vi "ThorlabsManager.vi"(3 "error in (no error)":errorcluster caption="错误输入（无错误）", 4 "Input":T3, 5 "ref_in":T1) -> (0 "error out":errorcluster caption="错误输出", 1 "Output":T3, 2 "ref_out":T1)   [LabVIEW 2012]
panel:
  in  "ref_type":T2
  in  "MG17Motor 6":refnum<k7>(container)
  in  "MG17Motor 5":refnum<k7>(container)
  in  "MG17Motor 4":refnum<k7>(container)
  in  "MG17Motor 3":refnum<k7>(container)
  in  "MG17Motor 2":refnum<k7>(container)
  in  "MG17Motor":refnum<k7>(container)
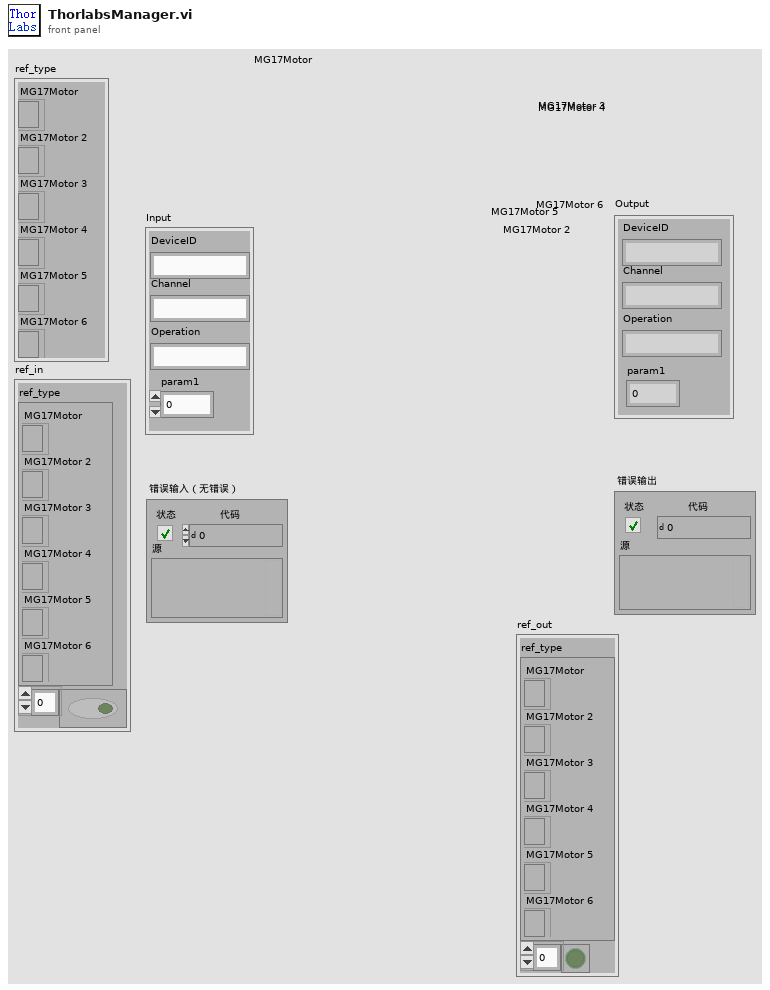
[diagram p1: front panel]
types:
  T1 = cluster{"ref_type":cluster{"MG17Motor":refnum<k7>, "MG17Motor 2":refnum<k7>, "MG17Motor 3":refnum<k7>, "MG17Motor 4":refnum<k7>, "MG17Motor 5":refnum<k7>, "MG17Motor 6":refnum<k7>}, bool[]}
  T2 = cluster{"MG17Motor":refnum<k7>, "MG17Motor 2":refnum<k7>, "MG17Motor 3":refnum<k7>, "MG17Motor 4":refnum<k7>, "MG17Motor 5":refnum<k7>, "MG17Motor 6":refnum<k7>}
  T3 = cluster{"DeviceID":string, "Channel":string, "param1":dbl, "Operation":string}
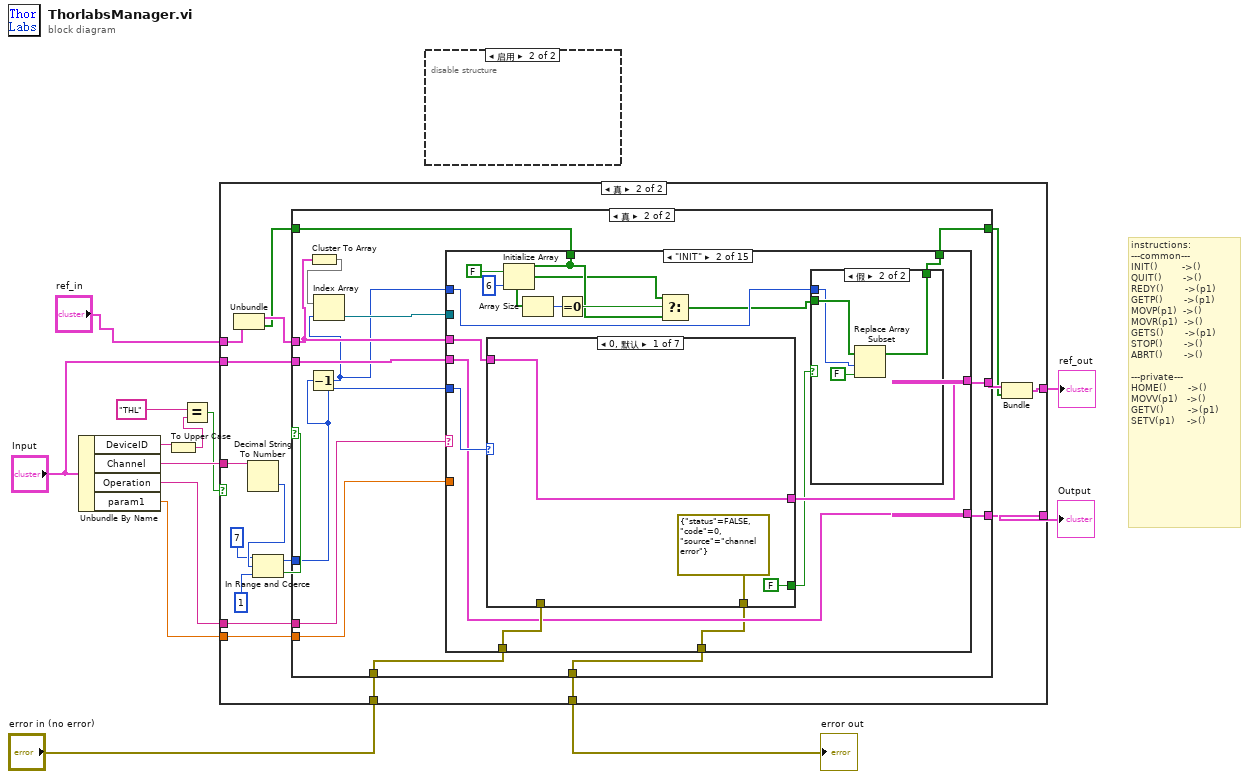
[diagram p0: block diagram]
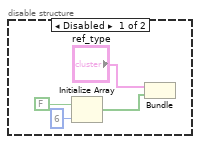
[diagram p2: hidden frame]
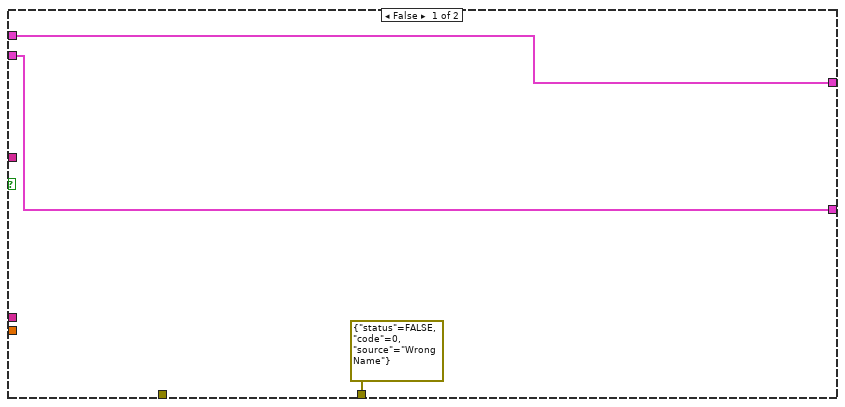
[diagram p3: hidden frame]
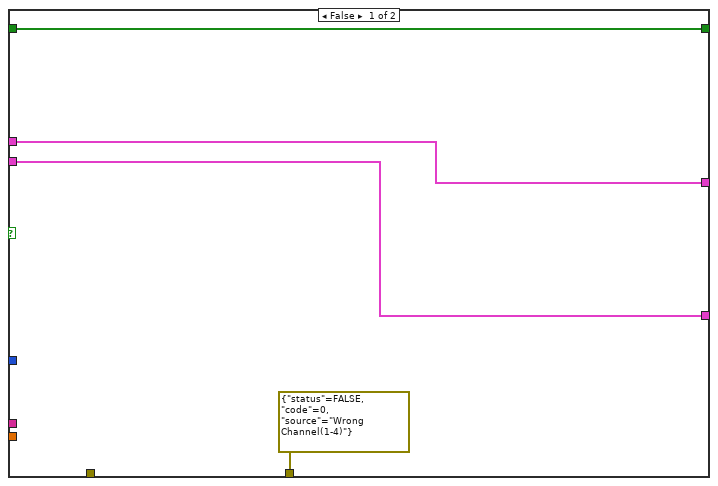
[diagram p4: hidden frame]
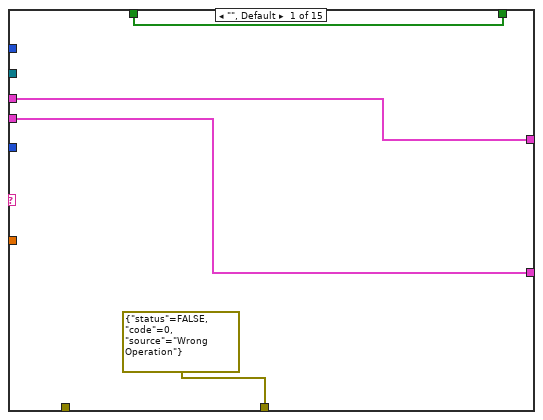
[diagram p5: hidden frame]
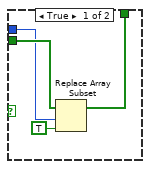
[diagram p6: hidden frame]
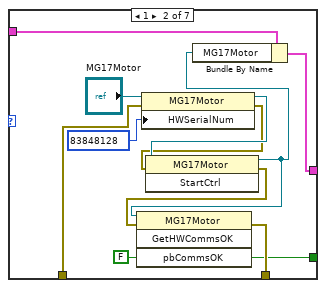
[diagram p7: hidden frame]
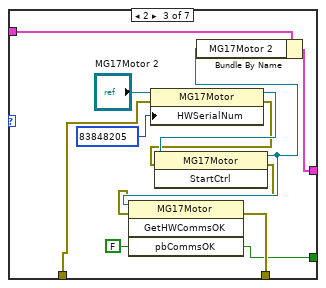
[diagram p8: hidden frame]
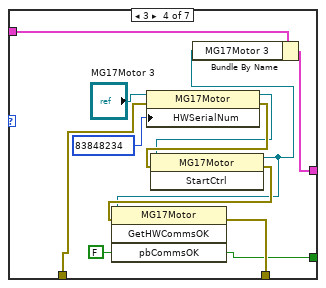
[diagram p9: hidden frame]
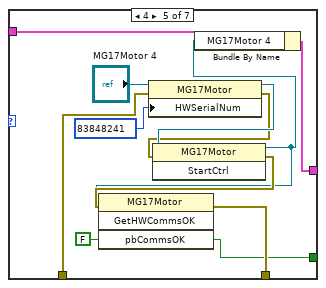
[diagram p10: hidden frame]
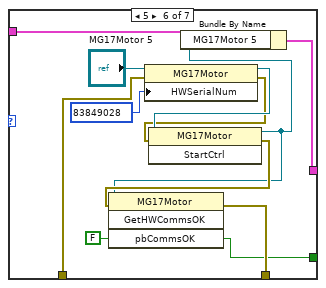
[diagram p11: hidden frame]
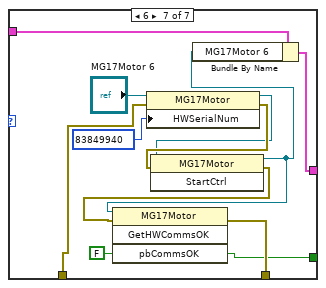
[diagram p12: hidden frame]
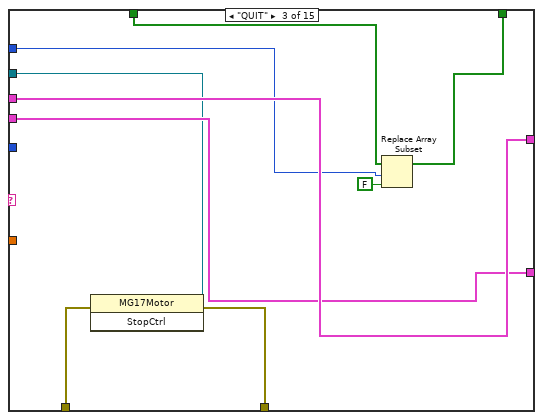
[diagram p13: hidden frame]
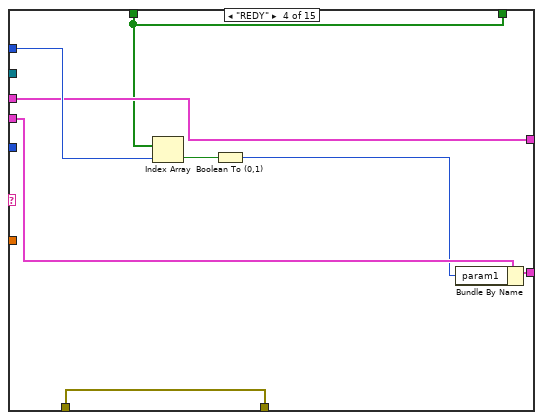
[diagram p14: hidden frame]
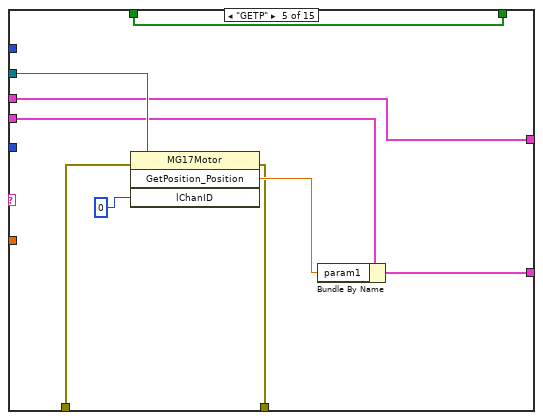
[diagram p15: hidden frame]
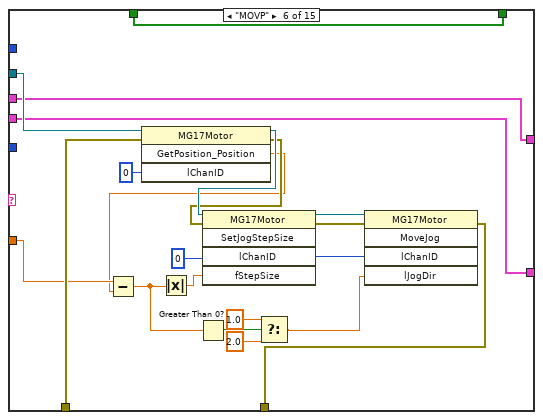
[diagram p16: hidden frame]
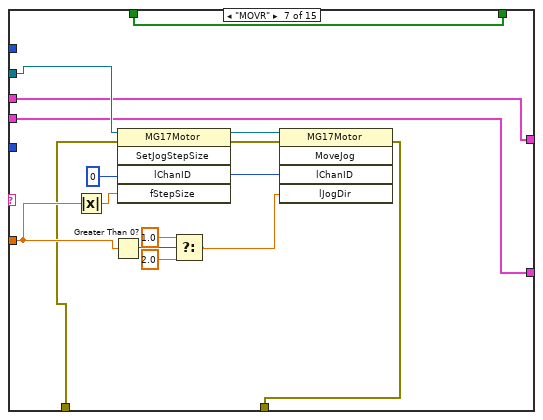
[diagram p17: hidden frame]
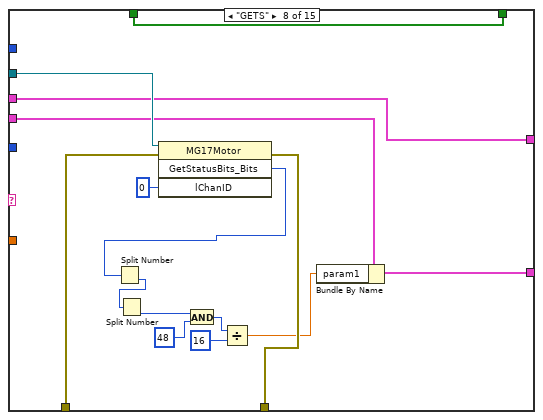
[diagram p18: hidden frame]
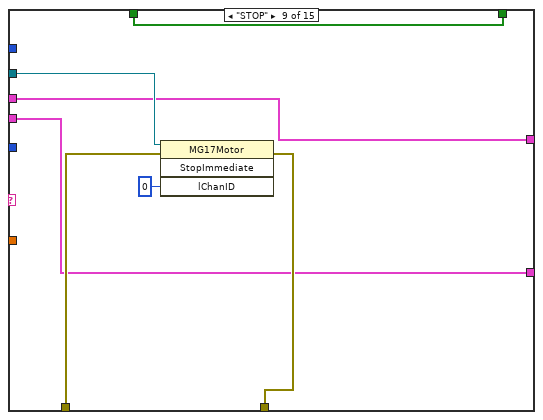
[diagram p19: hidden frame]
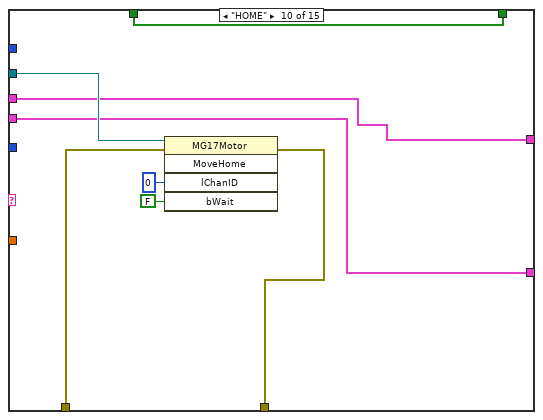
[diagram p20: hidden frame]
diagram:
  # "instructions:\n---common---\nINIT()        ->()\nQUIT()       ->()\nREDY()       ->(p1)\nGETP()       ->(p1)\nMOVP(p1)  ->()\nMOVR(p1)  ->()\nGETS()       ->(p1)\nSTOP()       ->()\nABRT()       ->()\n\n---private---\nHOME()       ->()\nMOVV(p1)   ->()\nGETV()        ->(p1)\nSETV(p1)    ->()"
  n1 = Unbundle By Name("Input") -> ("DeviceID"=w2:string, "Channel"=w12:string, "Operation"=w11:string, "param1"=w10:dbl)
  n2 = To Upper Case(1:w2) -> (0:w1:string)
  n3 = Equal?(x="THL", y=w1) -> (x = y?=w5:bool)
  n4 = case shown="真" w5 {
    tunnel: w12 -> [_ w34]
    tunnel: w11 -> [_ w28]
    tunnel: w10 -> [_ w27]
    tunnel: "error in (no error)" -> [_ w26]
    tunnel: [errorcluster {"status"=FALSE, "code"=0, "source"="Wrong Name"} ("error out") w25] -> w8
    tunnel: [w16 w24] -> w7
    tunnel: "ref_in" -> [w14 w22]
    tunnel: "Input" -> [w16 w23]
    tunnel: [w14 w17] -> w4
    frame False {
    }
    frame True {
      n5 = Unbundle(w22) -> ("ref_type"=w21:T2, w20:bool[])
      n6 = Decimal String To Number(string=w34) -> (number=w33:i32)  [unwired: 2 in, 1 out]
      n7 = In Range and Coerce(upper limit=7 ("上限"), x=w33, lower limit=1 ("下限")) -> (coerced(x)=w29:i32, In Range?=w30:bool)
      n8 = case shown="真" w30 {
        tunnel: w29 -> [_ w42]
        tunnel: w28 -> [_ w52]
        tunnel: w27 -> [_ w51]
        tunnel: w26 -> [_ w50]
        tunnel: [errorcluster {"status"=FALSE, "code"=0, "source"="Wrong Channel(1-4)"} ("error out") w49] -> w25
        tunnel: [w38 w48] -> w24
        tunnel: w21 -> [w36 w45]
        tunnel: w23 -> [w38 w47]
        tunnel: [w36 w46] -> w19
        tunnel: w20 -> [w35 w41]
        tunnel: [w35 w40] -> w18
        frame False {
        }
        frame True {
          n9 = Decrement(x=w42) -> (x-1=w39:i32)
          n10 = Cluster To Array(cluster=w45) -> (array=w44:refnum<k7>[])
          n11 = Index Array(array=w44, index=w39) -> (element=w43:refnum<k7>)
          n12 = case shown="\"INIT\"" w52 {
            tunnel: w42 -> [_ w72 _ _ _ _ _ _ _ _ _ _ _ _ _]
            tunnel: w51 -> [_ _ _ _ _ w189 w213 _ _ _ w253 _ w279 w283 w298]
            tunnel: w50 -> [_ w70 w164 w165 w174 w190 w211 w231 w238 w247 w257 w262 w275 w287 w296]
            tunnel: [errorcluster {"status"=FALSE, "code"=0, "source"="Wrong Operation"} ("error out") w67 w160 w165 w175 w185 w210 w232 w237 w246 w256 w261 w274 w288 w295] -> w49
            tunnel: [w56 w68 w162 w170 w179 w183 w209 w227 w235 w245 w254 w266 w278 w285 w293] -> w48
            tunnel: w45 -> [w54 w71 w163 w167 w177 w184 w208 w228 w236 w244 w255 w263 w277 w286 w294]
            tunnel: w47 -> [w56 w68 w162 w169 w178 w183 w209 w229 w235 w245 w254 w265 w278 w285 w293]
            tunnel: [w54 w69 w163 w167 w177 w184 w208 w228 w236 w244 w255 w263 w277 w286 w294] -> w46
            tunnel: w43 -> [_ _ w161 _ w181 w193 w212 w233 w240 w248 w258 w269 w281 w291 w297]
            tunnel: w41 -> [w53 w62 w158 w166 w173 w182 w207 w219 w234 w242 w260 w267 w276 w284 w292]
            tunnel: [w53 w65 w157 w166 w173 w182 w207 w219 w234 w242 w260 w267 w276 w284 w292] -> w40
            tunnel: w39 -> [_ w66 w159 w172 _ _ _ _ _ _ _ _ _ _ _]
            frame "", Default {
            }
            frame "INIT" {
              n13 = case shown="0, 默认" w72 {
                tunnel: w71 -> [w82 w91 w103 w115 w127 w139 w150]
                tunnel: w70 -> [_ w90 w101 w113 w125 w137 w151]
                tunnel: [errorcluster {"status"=FALSE, "code"=0, "source"="channel error"} ("错误输出") w86 w98 w110 w122 w134 w146] -> w67
                tunnel: [w82 w89 w102 w114 w126 w138 w149] -> w69
                tunnel: [FALSE ("pbCommsOK") w84 w96 w108 w120 w132 w144] -> w57
                frame 0, Default {
                }
                frame 1 {
                  n14 = property class="MG17Motor"(reference="MG17Motor", error in=w90, "HWSerialNum"=83848128) -> (reference out=w94:refnum<k7>, error out=w92:errorcluster)
                  n15 = invoke class="MG17Motor" method="StartCtrl"(reference=w94, error in=w92) -> (reference out=w88:refnum<k7>, error out=w87:errorcluster)  [unwired: 1 in, 1 out]
                  n16 = invoke class="MG17Motor" method="GetHWCommsOK"(reference=w88, error in=w87, "pbCommsOK"=FALSE ("pbStarted")) -> (error out=w86:errorcluster, "pbCommsOK"=w84:bool)  [unwired: 1 in, 2 out]
                  n17 = Bundle By Name(cluster=w91, "MG17Motor"=w88) -> (w89:T2)
                }
                frame 2 {
                  n18 = property class="MG17Motor"(reference="MG17Motor 2", error in=w101, "HWSerialNum"=83848205) -> (reference out=w106:refnum<k7>, error out=w104:errorcluster)
                  n19 = invoke class="MG17Motor" method="StartCtrl"(reference=w106, error in=w104) -> (reference out=w100:refnum<k7>, error out=w99:errorcluster)  [unwired: 1 in, 1 out]
                  n20 = invoke class="MG17Motor" method="GetHWCommsOK"(reference=w100, error in=w99, "pbCommsOK"=FALSE ("pbStarted")) -> (error out=w98:errorcluster, "pbCommsOK"=w96:bool)  [unwired: 1 in, 2 out]
                  n21 = Bundle By Name(cluster=w103, "MG17Motor 2"=w100) -> (w102:T2)
                }
                frame 3 {
                  n22 = property class="MG17Motor"(reference="MG17Motor 3", error in=w113, "HWSerialNum"=83848234) -> (reference out=w117:refnum<k7>, error out=w119:errorcluster)
                  n23 = invoke class="MG17Motor" method="StartCtrl"(reference=w117, error in=w119) -> (reference out=w111:refnum<k7>, error out=w112:errorcluster)  [unwired: 1 in, 1 out]
                  n24 = invoke class="MG17Motor" method="GetHWCommsOK"(reference=w111, error in=w112, "pbCommsOK"=FALSE ("pbStarted")) -> (error out=w110:errorcluster, "pbCommsOK"=w108:bool)  [unwired: 1 in, 2 out]
                  n25 = Bundle By Name(cluster=w115, "MG17Motor 3"=w111) -> (w114:T2)
                }
                frame 4 {
                  n26 = property class="MG17Motor"(reference="MG17Motor 4", error in=w125, "HWSerialNum"=83848241) -> (reference out=w130:refnum<k7>, error out=w128:errorcluster)
                  n27 = invoke class="MG17Motor" method="StartCtrl"(reference=w130, error in=w128) -> (reference out=w123:refnum<k7>, error out=w124:errorcluster)  [unwired: 1 in, 1 out]
                  n28 = invoke class="MG17Motor" method="GetHWCommsOK"(reference=w123, error in=w124, "pbCommsOK"=FALSE ("pbStarted")) -> (error out=w122:errorcluster, "pbCommsOK"=w120:bool)  [unwired: 1 in, 2 out]
                  n29 = Bundle By Name(cluster=w127, "MG17Motor 4"=w123) -> (w126:T2)
                }
                frame 5 {
                  n30 = property class="MG17Motor"(reference="MG17Motor 5", error in=w137, "HWSerialNum"=83849028) -> (reference out=w142:refnum<k7>, error out=w140:errorcluster)
                  n31 = invoke class="MG17Motor" method="StartCtrl"(reference=w142, error in=w140) -> (reference out=w135:refnum<k7>, error out=w136:errorcluster)  [unwired: 1 in, 1 out]
                  n32 = invoke class="MG17Motor" method="GetHWCommsOK"(reference=w135, error in=w136, "pbCommsOK"=FALSE ("pbStarted")) -> (error out=w134:errorcluster, "pbCommsOK"=w132:bool)  [unwired: 1 in, 2 out]
                  n33 = Bundle By Name(cluster=w139, "MG17Motor 5"=w135) -> (w138:T2)
                }
                frame 6 {
                  n34 = property class="MG17Motor"(reference="MG17Motor 6", error in=w151, "HWSerialNum"=83849940) -> (reference out=w153:refnum<k7>, error out=w155:errorcluster)
                  n35 = invoke class="MG17Motor" method="StartCtrl"(reference=w153, error in=w155) -> (reference out=w147:refnum<k7>, error out=w148:errorcluster)  [unwired: 1 in, 1 out]
                  n36 = invoke class="MG17Motor" method="GetHWCommsOK"(reference=w147, error in=w148, "pbCommsOK"=FALSE ("pbStarted")) -> (error out=w146:errorcluster, "pbCommsOK"=w144:bool)  [unwired: 1 in, 2 out]
                  n37 = Bundle By Name(cluster=w150, "MG17Motor 6"=w147) -> (w149:T2)
                }
              }
              n38 = Initialize Array(FALSE, 6 ("维数大小")) -> (w58:bool[])
              n39 = Array Size(array=w62) -> (size(s)=w64:i32)
              n40 = Equal To 0?(x=w64) -> (x = 0?=w63:bool)
              n41 = Select(t=w58, s=w63, f=w62) -> (s? t:f=w61:bool[])
              n42 = case shown="假" w57 {
                tunnel: w61 -> [w76 w79]
                tunnel: w66 -> [w75 w78]
                tunnel: [w73 w77] -> w65
                frame True {
                  n43 = Replace Array Subset(array=w76, new element=TRUE ("新元素/子数组"), index=w75) -> (w73:bool[])
                }
                frame False {
                  n44 = Replace Array Subset(array=w79, new element=FALSE ("新元素/子数组"), index=w78) -> (w77:bool[])
                }
              }
            }
            frame "QUIT" {
              n45 = invoke class="MG17Motor" method="StopCtrl"(reference=w161, error in=w164) -> (error out=w160:errorcluster)  [unwired: 1 in, 2 out]
              n46 = Replace Array Subset(array=w158, new element=FALSE ("新元素/子数组"), index=w159) -> (w157:bool[])
            }
            frame "REDY" {
              n47 = Index Array(array=w166, index=w172) -> (element=w171:bool)
              n48 = Boolean To (0,1)(Boolean=w171) -> (0, 1=w168:i16)
              n49 = Bundle By Name(cluster=w169, "param1"=w168) -> (w170:T3)
            }
            frame "GETP" {
              n50 = invoke class="MG17Motor" method="GetPosition_Position"(reference=w181, error in=w174, "lChanID"=0) -> (error out=w175:errorcluster, "GetPosition_Position"=w176:sgl)  [unwired: 1 in, 2 out]
              n51 = Bundle By Name(cluster=w178, "param1"=w176) -> (w179:T3)
            }
            frame "MOVP" {
              n52 = invoke class="MG17Motor" method="GetPosition_Position"(reference=w193, error in=w190, "lChanID"=0) -> (reference out=w192:refnum<k7>, error out=w191:errorcluster, "GetPosition_Position"=w188:sgl)  [unwired: 1 in, 1 out]
              n53 = Subtract(x=w189, y=w188) -> (x-y=w186:dbl)
              n54 = Absolute Value(x=w186) -> (abs(x)=w195:dbl)
              n55 = Greater Than 0?(x=w186) -> (x > 0?=w199:bool)
              n56 = invoke class="MG17Motor" method="SetJogStepSize"(reference=w192, error in=w191, "lChanID"=0, "fStepSize"=w195) -> (reference out=w198:refnum<k7>, error out=w197:errorcluster, "lChanID"=w196:i32)  [unwired: 1 in, 2 out]
              n57 = Select(t=1.0, s=w199, f=2.0) -> (s? t:f=w200:dbl)
              n58 = invoke class="MG17Motor" method="MoveJog"(reference=w198, error in=w197, "lChanID"=w196, "lJogDir"=w200) -> (error out=w185:errorcluster)  [unwired: 1 in, 4 out]
            }
            frame "MOVR" {
              n59 = Absolute Value(x=w213) -> (abs(x)=w217:dbl)
              n60 = Greater Than 0?(x=w213) -> (x > 0?=w206:bool)
              n61 = invoke class="MG17Motor" method="SetJogStepSize"(reference=w212, error in=w211, "lChanID"=0, "fStepSize"=w217) -> (reference out=w214:refnum<k7>, error out=w215:errorcluster, "lChanID"=w216:i32)  [unwired: 1 in, 2 out]
              n62 = Select(t=1.0, s=w206, f=2.0) -> (s? t:f=w205:dbl)
              n63 = invoke class="MG17Motor" method="MoveJog"(reference=w214, error in=w215, "lChanID"=w216, "lJogDir"=w205) -> (error out=w210:errorcluster)  [unwired: 1 in, 4 out]
            }
            frame "GETS" {
              n64 = invoke class="MG17Motor" method="GetStatusBits_Bits"(reference=w233, error in=w231, "lChanID"=0) -> (error out=w232:errorcluster, "GetStatusBits_Bits"=w226:i32)  [unwired: 1 in, 2 out]
              n65 = Split Number(x=w226) -> (lo(x)=w225:u16)  [unwired: 1 out]
              n66 = Split Number(x=w225) -> (lo(x)=w224:u8)  [unwired: 1 out]
              n67 = And(x=w224, y=u8 48) -> (x .and. y?=w222:u8)
              n68 = Divide(x=w222, y=u8 16) -> (x/y=w220:dbl)
              n69 = Bundle By Name(cluster=w229, "param1"=w220) -> (w227:T3)
            }
            frame "STOP" {
              n70 = invoke class="MG17Motor" method="StopImmediate"(reference=w240, error in=w238, "lChanID"=0) -> (error out=w237:errorcluster)  [unwired: 1 in, 3 out]
            }
            frame "HOME" {
              n71 = invoke class="MG17Motor" method="MoveHome"(reference=w248, error in=w247, "lChanID"=0, "bWait"=FALSE) -> (error out=w246:errorcluster)  [unwired: 1 in, 4 out]
            }
            frame "MOVV" {
              n72 = Greater Than 0?(x=w253) -> (x > 0?=w252:bool)
              n73 = Select(t=2.0, s=w252, f=1.0) -> (s? t:f=w251:dbl)
              n74 = invoke class="MG17Motor" method="MoveVelocity"(reference=w258, error in=w257, "lChanID"=0, "lDirection"=w251) -> (error out=w256:errorcluster)  [unwired: 1 in, 4 out]
            }
            frame "GETV" {
              n75 = invoke class="MG17Motor" method="GetVelParams_MaxVel"(reference=w269, error in=w262, "lChanID"=0) -> (error out=w261:errorcluster, "GetVelParams_MaxVel"=w264:sgl)  [unwired: 1 in, 2 out]
              n76 = Bundle By Name(cluster=w265, "param1"=w264) -> (w266:T3)
            }
            frame "SETV" {
              w270 = 0 ("lChanID")
              n77 = invoke class="MG17Motor" method="GetVelParams_Accn"(reference=w281, error in=w275, "lChanID"=0) -> (reference out=w280:refnum<k7>, error out=w273:errorcluster, "GetVelParams_Accn"=w271:sgl)  [unwired: 1 in, 1 out]
              n78 = invoke class="MG17Motor" method="SetVelParams"(reference=w280, error in=w273, "lChanID"=w270, "fMinVel"=w270, "fAccn"=w271, "fMaxVel"=w279) -> (error out=w274:errorcluster)  [unwired: 1 in, 6 out]
            }
            frame "MOVP_BAK" {
              n79 = invoke class="MG17Motor" method="MoveAbsoluteEx"(reference=w291, error in=w287, "lChanID"=0, "fAbsPosCh1"=w283, "fAbsPosCh2"=sgl 0.0, "bWait"=FALSE) -> (error out=w288:errorcluster)  [unwired: 1 in, 6 out]
            }
            frame "MOVR_BAK" {
              n80 = invoke class="MG17Motor" method="MoveRelativeEx"(reference=w297, error in=w296, "lChanID"=0, "fRelDistCh1"=w298, "fRelDistCh2"=sgl 0.0, "bWait"=FALSE) -> (error out=w295:errorcluster)  [unwired: 1 in, 6 out]
            }
          }
        }
      }
      n81 = Bundle("ref_type"=w19, w18) -> (w17:T1)  [unwired: 1 in]
    }
  }
  "Output" <- w7
  "error out" <- w8
  "ref_out" <- w4
  n82 = disable-structure shown="启用" {
    frame Disabled {
      n83 = Initialize Array(FALSE, 6 ("维数大小")) -> (w302:bool[])
      n84 = Bundle("ref_type"="ref_type", w302) -> ()  [unwired: 1 in, 1 out]
    }
    frame Enabled {
    }
  }
